vi "testCreateQueueTcpClientFromDds.vi"(8 "error in (no error)":errorcluster) -> (0 "error out":errorcluster)   [LabVIEW 2018]
doc: "Test the createQueueTcpClientFromDds.vi."
uses:
  src/TcpServerTel/TcpServerTel.lvclass
  src/TcpServerTel/TcpServerTel.lvclass/TcpServerTel.ctl
  <vilib>/addons/_JKI Toolkits/Caraya/classes/Assert/Assert Equal Type_Variant.vi
  <vilib>/addons/_JKI Toolkits/Caraya/classes/Test/Test.lvclass
  <vilib>/addons/_JKI Toolkits/Caraya/classes/Assert/Assert.lvclass
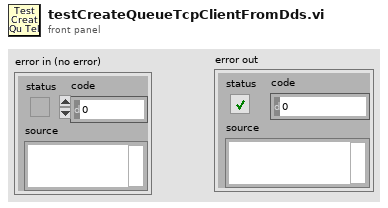
[diagram p1: front panel]
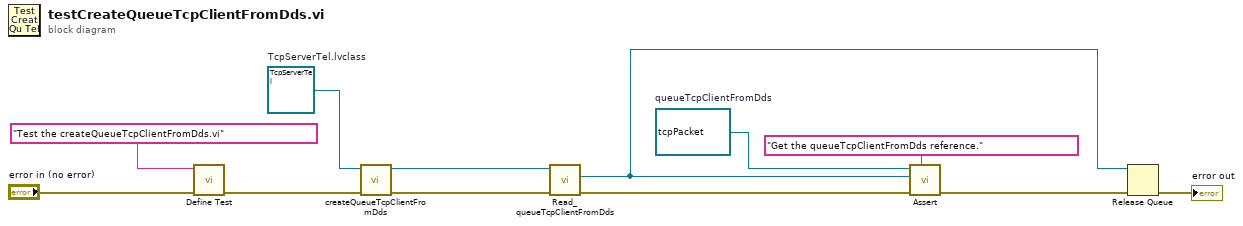
[diagram p0: block diagram]
diagram:
  w1 = refnum<queue> refnum  # queueTcpClientFromDds
  w8 = refnum<class "TcpServerTel.lvclass"> refnum  # TcpServerTel.lvclass
  n1 = call <vilib>:"Define Test.vi"("error in (no error)"="error in (no error)", "Label (VI Title)"="Test the createQueueTcpClientFromDds.vi") -> ("error out"=w7:errorcluster)  [unwired: 9 in]
  n2 = call "createQueueTcpClientFromDds.vi"("error in (no error)"=w7, "tcpServerTel in"=w8) -> ("error out"=w5:errorcluster, "tcpServerTel out"=w6:refnum<class "TcpServerTel.lvclass">)  [unwired: 8 in]
  n3 = call "Read_queueTcpClientFromDds.vi"("error in (no error)"=w5, "TcpServerTel in"=w6) -> ("error out"=w4:errorcluster, "queueTcpClientFromDds"=w2:refnum<queue>)  [unwired: 7 in, 1 out]
  n4 = call-poly <vilib>:"Assert.vi"("Label"="Get the queueTcpClientFromDds reference.", "error in (no error)"=w4, "Y"=w2, "X"=w1) -> ("error out"=w10:errorcluster)  [unwired: 7 in]
  n5 = Release Queue(queue=w2, error in (no error)=w10) -> (error out=→"error out":errorcluster)  [unwired: 1 in, 2 out]
